vi "Pre Launch Init.vi"(11 "Cam_SLM_Controller in":refnum<class "Cam_SLM_Controller.lvclass">) -> (0 "error out":errorcluster, 3 "Cam_SLM_Controller out":refnum<class "Cam_SLM_Controller.lvclass">)   [LabVIEW 2023, in "Cam_SLM_controller.lvlib" / "Cam_SLM_Controller.lvclass"]
doc: "(<B>Filename</B>: Actor Framework.lvlib:Actor.lvclass:Pre Launch Init.vi)\n\nDefines behavior that occurs after the Launch Nested Actor method is invoked but before the actor's Actor Core method begins running.\n\nBy default, this method does nothing. A descendant class may override it to define behavior."
uses:
  Cam_SLM_Controller.lvclass
  Cam_SLM_Controller.lvclass/Cam_SLM_Controller.ctl
  <vilib>/ActorFramework/Actor/Actor.lvclass
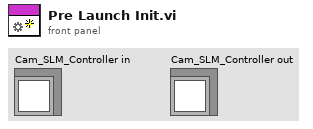
[diagram p1: front panel]
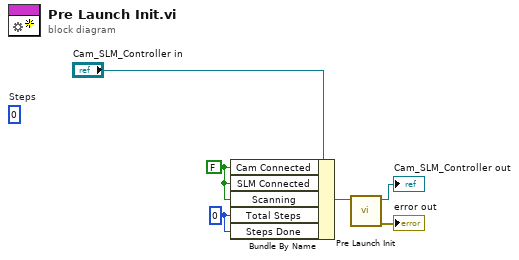
[diagram p0: block diagram]
diagram:
  w1 = u16 0 ("Total Steps")
  w2 = FALSE ("Cam Connected")
  (unwired) 0  # Steps
  n1 = Bundle By Name(cluster="Cam_SLM_Controller in", "Cam Connected"=w2, "SLM Connected"=w2, "Scanning"=w2, "Total Steps"=w1, "Steps Done"=w1) -> (w3:refnum<class "Cam_SLM_Controller.lvclass">)
  n2 = call-parent "Pre Launch Init.vi"("Actor in"=w3) -> ("error out"=→"error out":errorcluster, "Actor out"=→"Cam_SLM_Controller out":refnum<class "Cam_SLM_Controller.lvclass">)  [unwired: 9 in]
